vi "queryData.vi"(8 "error in (no error)":errorcluster, 10 "queries":T1, 11 "DomeCommunicator in":refnum<class "DomeCommunicator.lvclass">) -> (0 "error out":errorcluster, 1 "timeout":bool, 2 "response":string, 3 "DomeCommunicator out":refnum<class "DomeCommunicator.lvclass">)   [LabVIEW 2016, in "DomeCommunicator.lvclass"]
uses:
  DomeCommunicator.lvclass
  C:/Users/aanania/Documents/common_labview_tcpdevice/tcpDevice/tcpDevice.lvclass
  ComTypedefs/queries.ctl
  common_labview_tcpdevice/tcpDevice/tcpDevice.lvclass
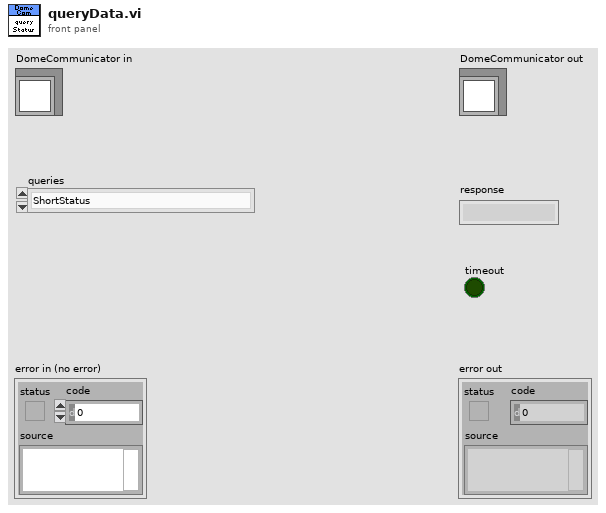
[diagram p1: front panel]
types:
  T1 = typedef "queries.ctl" = enum16{"ShortStatus", "FullEngineeringStatus", "RecallLastSavedConfiguration"}
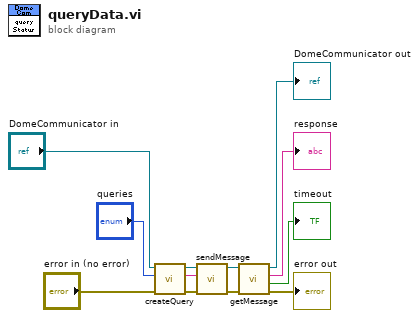
[diagram p0: block diagram]
diagram:
  n1 = call "createQuery.vi"("error in (no error)"="error in (no error)", "queries"="queries", "DomeCommunicator in"="DomeCommunicator in") -> ("error out"=w7:errorcluster, "query"=w1:string, "DomeCommunicator out"=w8:refnum<class "DomeCommunicator.lvclass">)  [unwired: 6 in]
  n2 = call "sendMessage.vi"("error in (no error)"=w7, "Message"=w1, "tcpDevice in"=w8) -> ("error out"=w6:errorcluster, "tcpDevice out"=w9:refnum<class "DomeCommunicator.lvclass">)  [unwired: 7 in]
  n3 = call "getMessage.vi"("error in (no error)"=w6, "tcpDevice in"=w9) -> ("error out"=→"error out":errorcluster, "timeout"=→"timeout":bool, "Message"=→"response":string, "tcpDevice out"=→"DomeCommunicator out":refnum<class "DomeCommunicator.lvclass">)  [unwired: 6 in]
